vi "constants.vi"(8 "error in (no error)":errorcluster) -> (0 "error out":errorcluster, 3 "DB connection File Path":path)   [LabVIEW 2011]
panel:
  in  "Testing":bool=TRUE
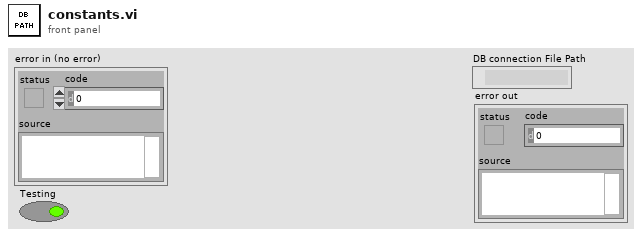
[diagram p1: front panel]
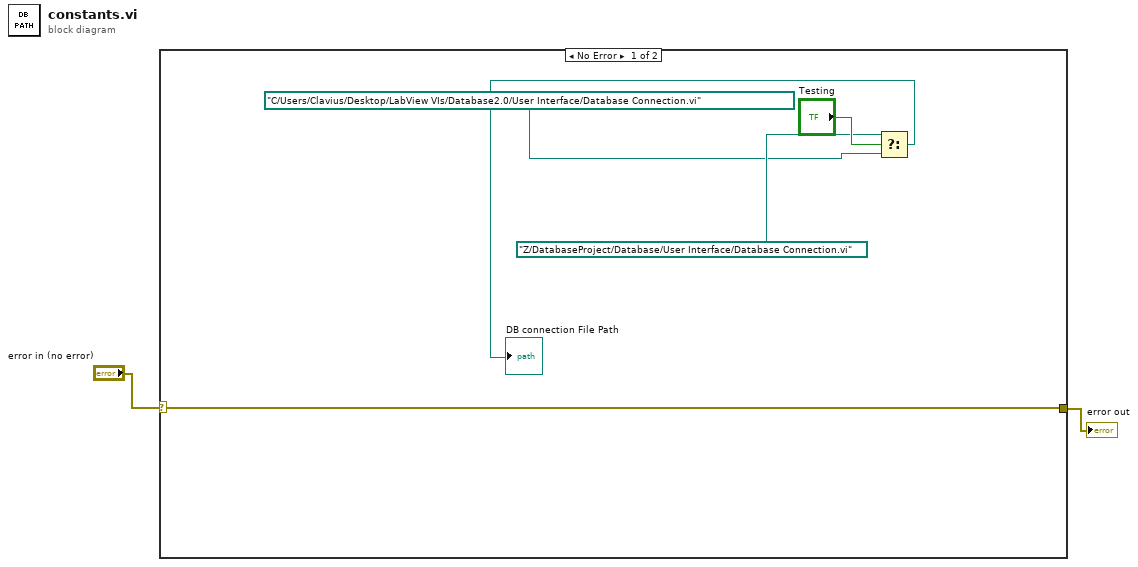
[diagram p0: block diagram]
diagram:
  n1 = case shown="No Error" "error in (no error)" {
    selector: "error in (no error)" -> [w3 w8]
    tunnel: [w3 w8] -> w2
    frame No Error {
      n2 = Select(t=path "Z:/DatabaseProject/Database/User Interface/Database Connection.vi", s="Testing", f=path "C:/Users/Clavius/Desktop/LabView VIs/Database2.0/User Interface/Database Connection.vi" ("vi path")) -> (s? t:f=→"DB connection File Path":path)
    }
    frame Error {
    }
  }
  "error out" <- w2
